vi "关键参数交互.vi"(9 "量程下拉列表":refnum<vi>, 10 "测量模式下拉列表":refnum<vi>, 11 "参数下拉列表":refnum<vi>) -> ()   [LabVIEW 2016, in "斯坦道总氮.lvlib"]
panel:
  out "总氮仪器参数":T1
  out "总磷仪器参数":T1
  out "x != y? 2":T2
  out "x != y?":T2
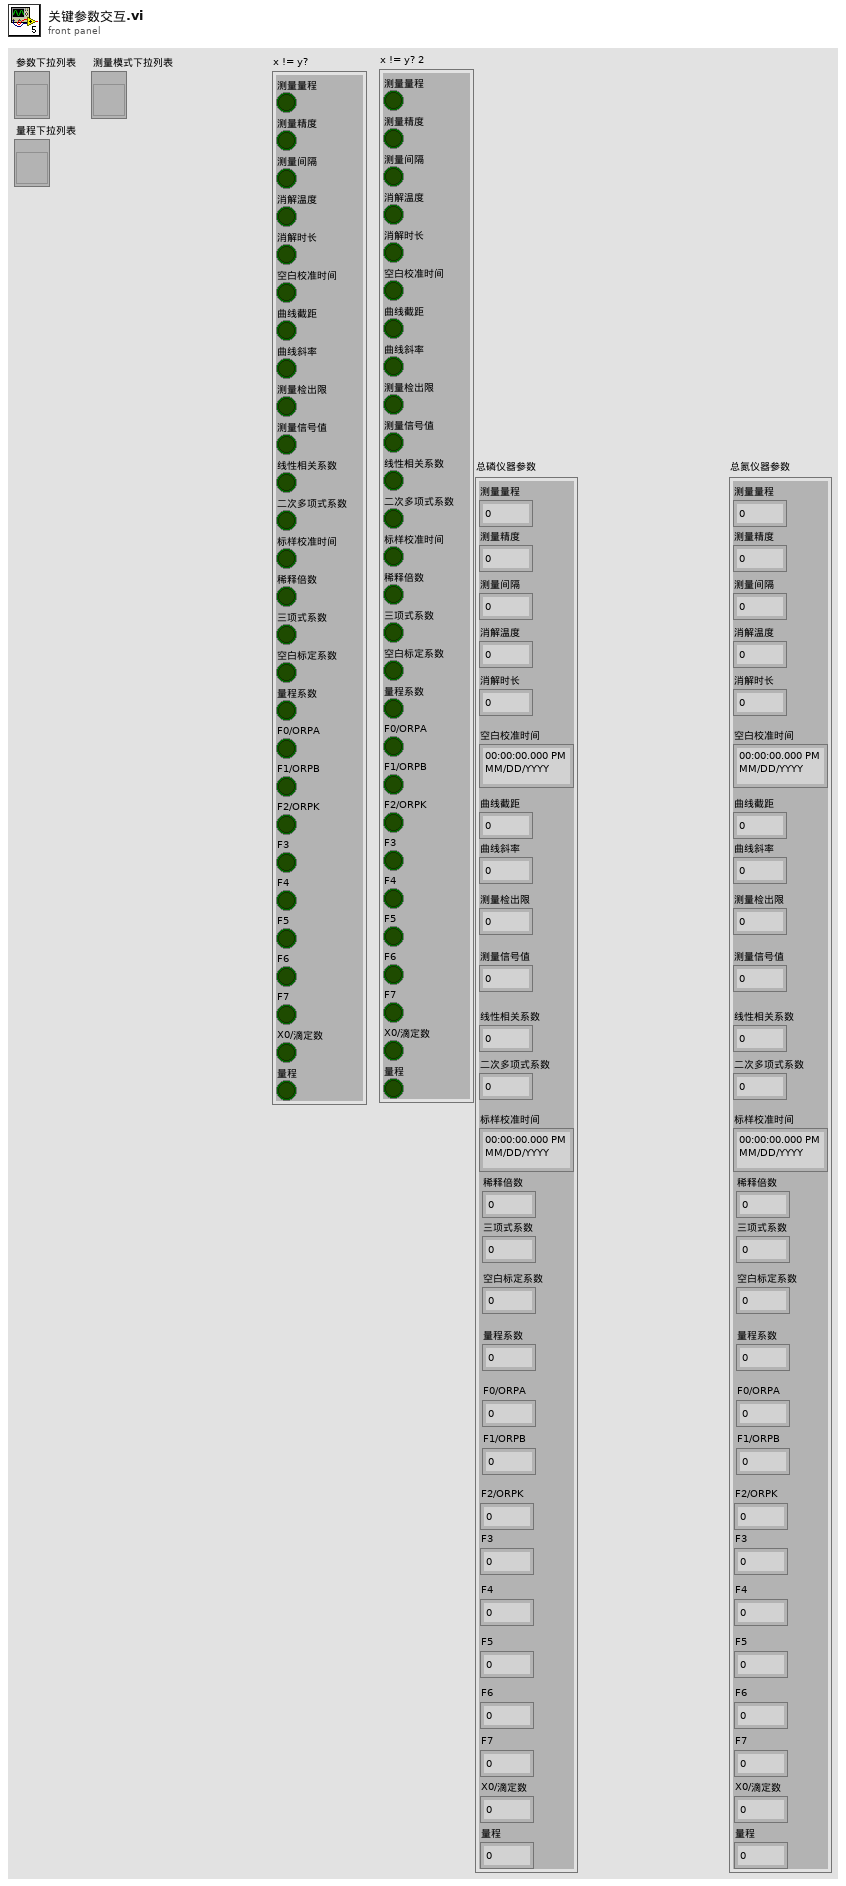
[diagram p1: front panel]
types:
  T1 = cluster{"测量量程":dbl, "测量精度":dbl, "测量间隔":dbl, "消解温度":dbl, "消解时长":dbl, "空白校准时间":timestamp, "曲线截距":dbl, "曲线斜率":dbl, "测量检出限":dbl, "测量信号值":dbl, "线性相关系数":dbl, "二次多项式系数":dbl, "标样校准时间":timestamp, "稀释倍数":dbl, "三项式系数":dbl, "空白标定系数":dbl, "量程系数":dbl, "F0/ORPA":dbl, "F1/ORPB":dbl, "F2/ORPK":dbl, "F3":dbl, "F4":dbl, "F5":dbl, "F6":dbl, "F7":dbl, "X0/滴定数":dbl, "量程":dbl}
  T2 = cluster{"测量量程":bool, "测量精度":bool, "测量间隔":bool, "消解温度":bool, "消解时长":bool, "空白校准时间":bool, "曲线截距":bool, "曲线斜率":bool, "测量检出限":bool, "测量信号值":bool, "线性相关系数":bool, "二次多项式系数":bool, "标样校准时间":bool, "稀释倍数":bool, "三项式系数":bool, "空白标定系数":bool, "量程系数":bool, "F0/ORPA":bool, "F1/ORPB":bool, "F2/ORPK":bool, "F3":bool, "F4":bool, "F5":bool, "F6":bool, "F7":bool, "X0/滴定数":bool, "量程":bool}
  T3 = cluster{"chose":string, "公式":cluster{"X^2":dbl, "X":dbl, "b":dbl}}
  T4 = cluster{"时间标识":timestamp, "设备":string, "日志信息":string, "流程参数":string}
  T5 = cluster{"[0]":bool, "[1]":bool, "[2]":bool, "[3]":bool, "[4]":bool, "[5]":bool, "[6]":bool, "[7]":bool, "[8]":bool, "[9]":bool, "[10]":bool, "[11]":bool, "[12]":bool, "[13]":bool, "[14]":bool, "[15]":bool, "[16]":bool, "[17]":bool, "[18]":bool, "[19]":bool, "[20]":bool, "[21]":bool, "[22]":bool, "[23]":bool, "[24]":bool, "[25]":bool, "[26]":bool}
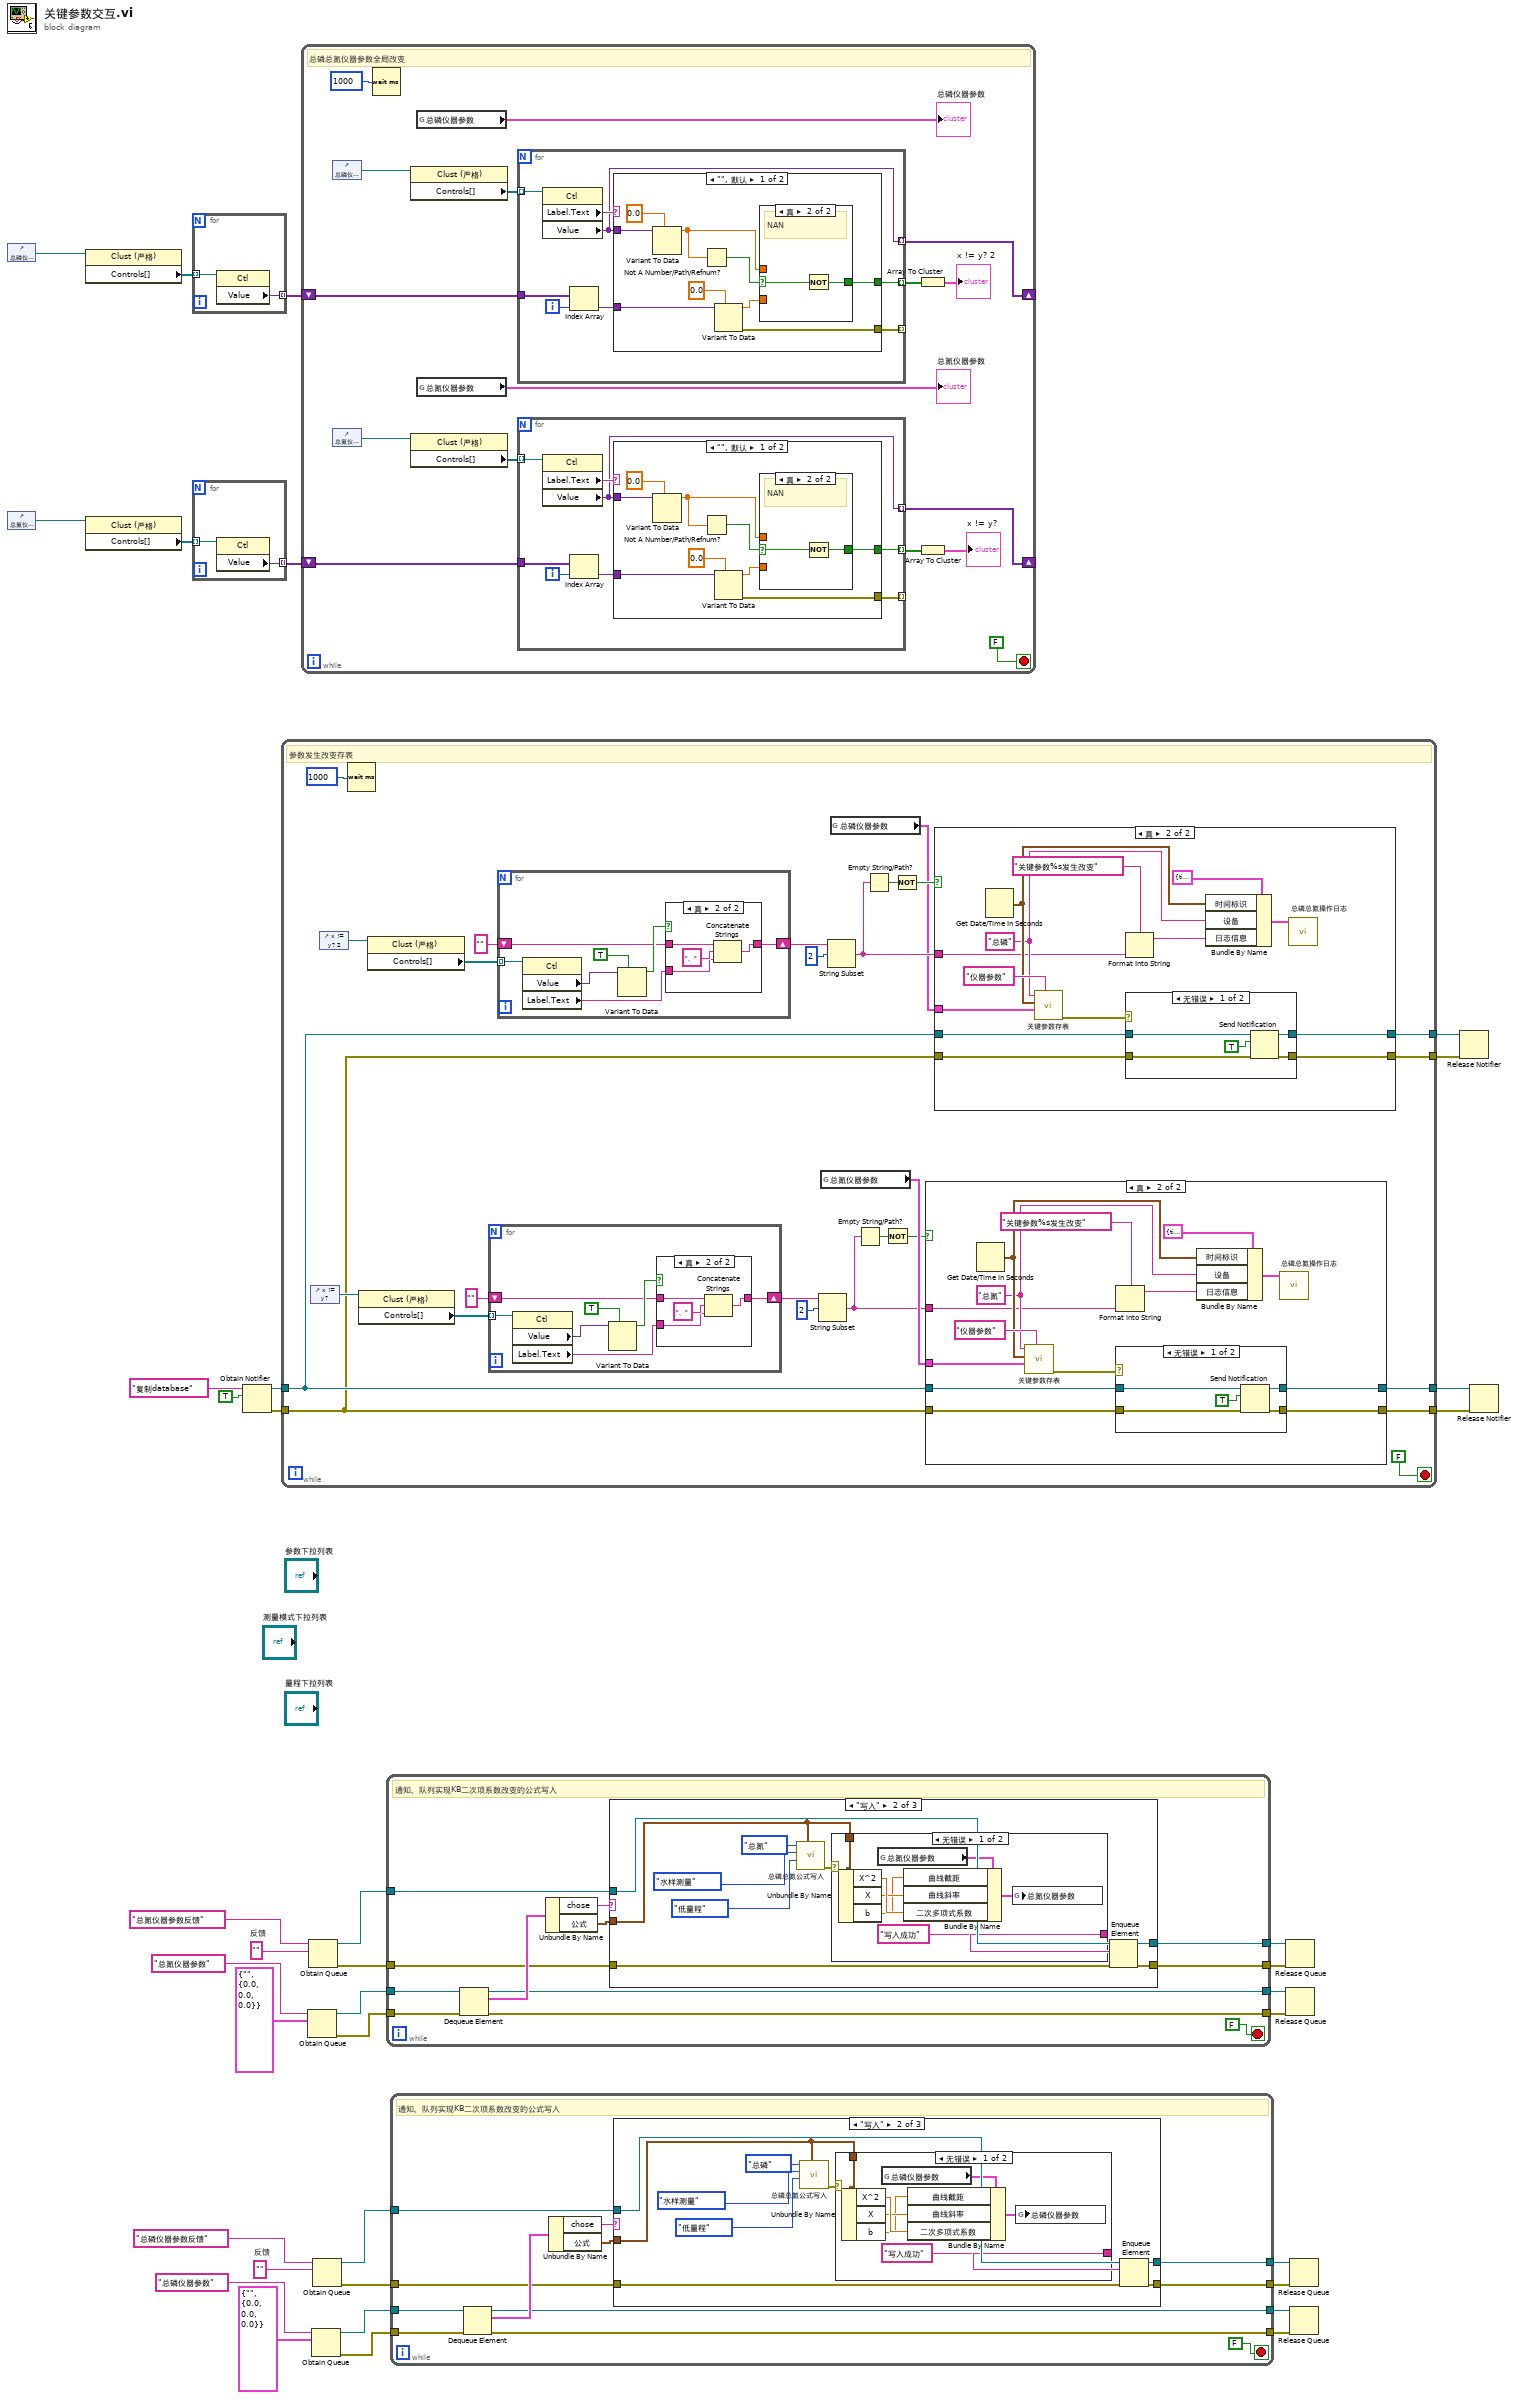
[diagram p0: block diagram]
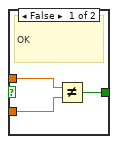
[diagram p2: hidden frame]
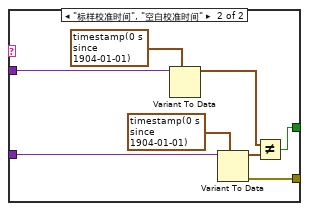
[diagram p3: hidden frame]
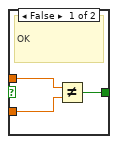
[diagram p4: hidden frame]
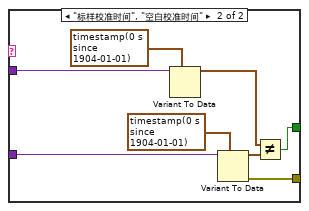
[diagram p5: hidden frame]
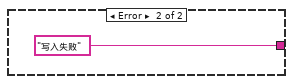
[diagram p7: hidden frame]
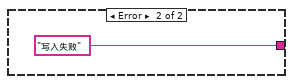
[diagram p10: hidden frame]
diagram:
  w15 = ""  # 反馈
  w32 = ""  # 反馈
  n1 = control-ref of="总磷仪器参数"() -> (w5:refnum<vi>)
  n2 = control-ref of="总氮仪器参数"() -> (w2:refnum<vi>)
  n3 = property class="Clust (严格)"(reference=w5) -> ("Controls[]"=w6:refnum<vi>[])  [unwired: 1 in, 2 out]
  n4 = property class="Clust (严格)"(reference=w2) -> ("Controls[]"=w3:refnum<vi>[])  [unwired: 1 in, 2 out]
  n5 = for {
    tunnel: w6 -> [w40] mode=indexing
    tunnel: [w39] -> w4 mode=indexing
    n6 = property class="Ctl"(reference=w40) -> ("Value"=w39:variant)  [unwired: 1 in, 2 out]
  }
  n7 = for {
    tunnel: w3 -> [w42] mode=indexing
    tunnel: [w41] -> w1 mode=indexing
    n8 = property class="Ctl"(reference=w42) -> ("Value"=w41:variant)  [unwired: 1 in, 2 out]
  }
  n9 = Obtain Notifier(name (unnamed)="复制database" ("名称（未命名）"), notification data type=TRUE) -> (notifier out=w24:refnum<notifier>, error out=w23:errorcluster)  [unwired: 2 in, 1 out]
  n10 = while {
    tunnel: w24 -> [w46]
    tunnel: w23 -> [w45]
    tunnel: [w64] -> w22
    tunnel: [w63] -> w21
    tunnel: [w44] -> w8
    tunnel: [w43] -> w7
    stop <- FALSE stop-if-true
    # "参数发生改变存表"
    n11 = control-ref of="x != y?"() -> (w66:refnum<vi>)
    n12 = control-ref of="x != y? 2"() -> (w48:refnum<vi>)
    n13 = Wait (ms)(milliseconds to wait=u32 1000 ("等待时间（毫秒）")) -> ()  [unwired: 1 out]
    n14 = property class="Clust (严格)"(reference=w66) -> ("Controls[]"=w59:refnum<vi>[])  [unwired: 1 in, 2 out]
    n15 = property class="Clust (严格)"(reference=w48) -> ("Controls[]"=w52:refnum<vi>[])  [unwired: 1 in, 2 out]
    n16 = for {
      tunnel: w59 -> [w110] mode=indexing
      shift-right: [w104] -> w61
      shift-left: "" -> [w106]
      n17 = property class="Ctl"(reference=w110) -> ("Value"=w108:variant, "Label.Text"=w105:string)  [unwired: 1 in, 2 out]
      n18 = Variant To Data(type=TRUE, Variant=w108) -> (data=w107:bool)  [unwired: 1 in, 1 out]
      n19 = case shown="真" w107 {
        tunnel: w106 -> [w111 w115]
        tunnel: w105 -> [_ w112]
        tunnel: [w111 w114] -> w104
        frame False {
        }
        frame True {
          n20 = Concatenate Strings(w115, "、", w112) -> (w114:string)
        }
      }
    }
    n21 = for {
      tunnel: w52 -> [w75] mode=indexing
      shift-right: [w69] -> w50
      shift-left: "" -> [w71]
      n22 = property class="Ctl"(reference=w75) -> ("Value"=w73:variant, "Label.Text"=w70:string)  [unwired: 1 in, 2 out]
      n23 = Variant To Data(type=TRUE, Variant=w73) -> (data=w72:bool)  [unwired: 1 in, 1 out]
      n24 = case shown="真" w72 {
        tunnel: w71 -> [w76 w80]
        tunnel: w70 -> [_ w77]
        tunnel: [w76 w79] -> w69
        frame False {
        }
        frame True {
          n25 = Concatenate Strings(w80, "、", w77) -> (w79:string)
        }
      }
    }
    n26 = String Subset(string=w61, offset (0)=2 ("偏移量(0)")) -> (substring=w56:string)  [unwired: 1 in]
    n27 = global read "总磷总氮断电保存全局变量.vi" "总氮仪器参数"() -> (w65:T1)
    n28 = String Subset(string=w50, offset (0)=2 ("偏移量(0)")) -> (substring=w55:string)  [unwired: 1 in]
    n29 = global read "总磷总氮断电保存全局变量.vi" "总磷仪器参数"() -> (w47:T1)
    n30 = Empty String/Path?(string/path=w56) -> (empty?=w58:bool)
    n31 = Empty String/Path?(string/path=w55) -> (empty?=w53:bool)
    n32 = Not(x=w58) -> (.not. x?=w57:bool)
    n33 = Not(x=w53) -> (.not. x?=w54:bool)
    n34 = case shown="真" w57 {
      tunnel: w65 -> [_ w130]
      tunnel: w56 -> [_ w124]
      tunnel: w46 -> [w117 w122]
      tunnel: w45 -> [w116 w121]
      tunnel: [w117 w119] -> w64
      tunnel: [w116 w118] -> w63
      frame False {
      }
      frame True {
        w126 = "总氮" ("仪器名称")
        n35 = Get Date/Time In Seconds() -> (seconds since 1Jan1904=w127:timestamp)
        n36 = call "关键参数存表.vi"("table"="仪器参数", "仪器参数"=w130, "datatime"=w127, "仪器名称"=w126) -> ("error out"=w120:errorcluster)  [unwired: 7 in]
        n37 = Format Into String(format string="关键参数%s发生改变" ("格式字符串"), w124) -> (resulting string=w123:string)  [unwired: 2 in, 1 out]
        n38 = case shown="无错误" w120 {
          tunnel: w122 -> [w136 w138]
          tunnel: w121 -> [w135 w137]
          tunnel: [w133 w138] -> w119
          tunnel: [w132 w137] -> w118
          frame No Error {
            n39 = Send Notification(notification=TRUE ("通知"), notifier=w136, error in (no error)=w135) -> (notifier out=w133:refnum<notifier>, error out=w132:errorcluster)
          }
          frame Error {
          }
        }
        n40 = Bundle By Name(cluster=T4 {"时间标识"=timestamp(0 s since 1904-01-01), "设备"="", "日志信息"="", "流程参数"=""} ("data in"), "时间标识"=w127, "设备"=w126, "日志信息"=w123) -> (w128:T4)
        n41 = call "总磷总氮操作日志.vi"("data in"=w128) -> ()  [unwired: 11 in]
      }
    }
    n42 = case shown="真" w54 {
      tunnel: w47 -> [_ w95]
      tunnel: w55 -> [_ w89]
      tunnel: w46 -> [w82 w87]
      tunnel: w45 -> [w81 w86]
      tunnel: [w82 w84] -> w44
      tunnel: [w81 w83] -> w43
      frame False {
      }
      frame True {
        w91 = "总磷" ("仪器名称")
        n43 = Get Date/Time In Seconds() -> (seconds since 1Jan1904=w92:timestamp)
        n44 = call "关键参数存表.vi"("table"="仪器参数", "仪器参数"=w95, "datatime"=w92, "仪器名称"=w91) -> ("error out"=w85:errorcluster)  [unwired: 7 in]
        n45 = Format Into String(format string="关键参数%s发生改变" ("格式字符串"), w89) -> (resulting string=w88:string)  [unwired: 2 in, 1 out]
        n46 = case shown="无错误" w85 {
          tunnel: w87 -> [w101 w103]
          tunnel: w86 -> [w100 w102]
          tunnel: [w98 w103] -> w84
          tunnel: [w97 w102] -> w83
          frame No Error {
            n47 = Send Notification(notification=TRUE ("通知"), notifier=w101, error in (no error)=w100) -> (notifier out=w98:refnum<notifier>, error out=w97:errorcluster)
          }
          frame Error {
          }
        }
        n48 = Bundle By Name(cluster=T4 {"时间标识"=timestamp(0 s since 1904-01-01), "设备"="", "日志信息"="", "流程参数"=""} ("data in"), "时间标识"=w92, "设备"=w91, "日志信息"=w88) -> (w93:T4)
        n49 = call "总磷总氮操作日志.vi"("data in"=w93) -> ()  [unwired: 11 in]
      }
    }
  }
  n50 = while {
    shift-right: [w148] -> _
    shift-left: w4 -> [w149]
    shift-right: [w139] -> _
    shift-left: w1 -> [w140]
    stop <- FALSE stop-if-true
    # "总磷总氮仪器参数全局改变"
    n51 = control-ref of="总磷仪器参数"() -> (w154:refnum<vi>)
    n52 = control-ref of="总氮仪器参数"() -> (w141:refnum<vi>)
    n53 = Wait (ms)(milliseconds to wait=u32 1000 ("等待时间（毫秒）")) -> ()  [unwired: 1 out]
    n54 = property class="Clust (严格)"(reference=w154) -> ("Controls[]"=w151:refnum<vi>[])  [unwired: 1 in, 2 out]
    n55 = property class="Clust (严格)"(reference=w141) -> ("Controls[]"=w143:refnum<vi>[])  [unwired: 1 in, 2 out]
    n56 = global read "总磷总氮断电保存全局变量.vi" "总磷仪器参数"() -> (→"总磷仪器参数":T1)
    n57 = global read "总磷总氮断电保存全局变量.vi" "总氮仪器参数"() -> (→"总氮仪器参数":T1)
    n58 = for {
      tunnel: w151 -> [w192] mode=indexing
      tunnel: [w190] -> w150 mode=indexing
      tunnel: [w188] -> _ mode=indexing
      tunnel: w149 -> [w187]
      tunnel: [w189] -> w148 mode=indexing
      i -> [w186]
      n59 = property class="Ctl"(reference=w192) -> ("Label.Text"=w191:string, "Value"=w189:variant)  [unwired: 1 in, 2 out]
      n60 = Index Array(array=w187, index=w186) -> (element=w185:variant)
      n61 = case shown="\"\", 默认" w191 {
        tunnel: w189 -> [w201 w214]
        tunnel: [w195 w208] -> w190
        tunnel: w185 -> [w198 w211]
        tunnel: [w197 w207] -> w188
        frame "", Default {
          n62 = Variant To Data(type=0.0 ("测量检出限"), Variant=w201) -> (data=w194:dbl)  [unwired: 1 in, 1 out]
          n63 = Not A Number/Path/Refnum?(number/path/refnum=w194) -> (NaN/Path/Refnum?=w196:bool)
          n64 = Variant To Data(type=0.0 ("测量检出限"), Variant=w198) -> (data=w193:dbl, error out=w197:errorcluster)  [unwired: 1 in]
          n65 = case shown="真" w196 {
            selector: w196 -> [_ w206]
            tunnel: [w202 w205] -> w195
            tunnel: w194 -> [w204 _]
            tunnel: w193 -> [w203 _]
            frame False {
              # "OK"
              n66 = Not Equal?(x=w204, y=w203) -> (x != y?=w202:bool)
            }
            frame True {
              # "NAN"
              n67 = Not(x=w206) -> (.not. x?=w205:bool)
            }
          }
        }
        frame "标样校准时间", "空白校准时间" {
          n68 = Variant To Data(type=timestamp(0 s since 1904-01-01), Variant=w214) -> (data=w210:timestamp)  [unwired: 1 in, 1 out]
          n69 = Variant To Data(type=timestamp(0 s since 1904-01-01), Variant=w211) -> (data=w209:timestamp, error out=w207:errorcluster)  [unwired: 1 in]
          n70 = Not Equal?(x=w210, y=w209) -> (x != y?=w208:bool)
        }
      }
    }
    n71 = for {
      tunnel: w143 -> [w162] mode=indexing
      tunnel: [w160] -> w144 mode=indexing
      tunnel: [w158] -> _ mode=indexing
      tunnel: w140 -> [w157]
      tunnel: [w159] -> w139 mode=indexing
      i -> [w156]
      n72 = property class="Ctl"(reference=w162) -> ("Label.Text"=w161:string, "Value"=w159:variant)  [unwired: 1 in, 2 out]
      n73 = Index Array(array=w157, index=w156) -> (element=w155:variant)
      n74 = case shown="\"\", 默认" w161 {
        tunnel: w159 -> [w171 w184]
        tunnel: [w165 w178] -> w160
        tunnel: w155 -> [w168 w181]
        tunnel: [w167 w177] -> w158
        frame "", Default {
          n75 = Variant To Data(type=0.0 ("测量检出限"), Variant=w171) -> (data=w164:dbl)  [unwired: 1 in, 1 out]
          n76 = Not A Number/Path/Refnum?(number/path/refnum=w164) -> (NaN/Path/Refnum?=w166:bool)
          n77 = Variant To Data(type=0.0 ("测量检出限"), Variant=w168) -> (data=w163:dbl, error out=w167:errorcluster)  [unwired: 1 in]
          n78 = case shown="真" w166 {
            selector: w166 -> [_ w176]
            tunnel: [w172 w175] -> w165
            tunnel: w164 -> [w174 _]
            tunnel: w163 -> [w173 _]
            frame False {
              # "OK"
              n79 = Not Equal?(x=w174, y=w173) -> (x != y?=w172:bool)
            }
            frame True {
              # "NAN"
              n80 = Not(x=w176) -> (.not. x?=w175:bool)
            }
          }
        }
        frame "标样校准时间", "空白校准时间" {
          n81 = Variant To Data(type=timestamp(0 s since 1904-01-01), Variant=w184) -> (data=w180:timestamp)  [unwired: 1 in, 1 out]
          n82 = Variant To Data(type=timestamp(0 s since 1904-01-01), Variant=w181) -> (data=w179:timestamp, error out=w177:errorcluster)  [unwired: 1 in]
          n83 = Not Equal?(x=w180, y=w179) -> (x != y?=w178:bool)
        }
      }
    }
    n84 = Array To Cluster(array=w150) -> (cluster=→"x != y? 2":T5)
    n85 = Array To Cluster(array=w144) -> (cluster=→"x != y?":T5)
  }
  n86 = Obtain Queue(name (unnamed)="总氮仪器参数" ("名称（未命名）"), element data type=T3 {"chose"="", "公式"={"X^2"=0.0, "X"=0.0, "b"=0.0}}) -> (queue out=w28:refnum<queue>, error out=w27:errorcluster)  [unwired: 3 in, 1 out]
  n87 = Obtain Queue(name (unnamed)="总氮仪器参数反馈" ("名称（未命名）"), element data type=w32) -> (queue out=w33:refnum<queue>, error out=w31:errorcluster)  [unwired: 3 in, 1 out]
  n88 = Obtain Queue(name (unnamed)="总磷仪器参数" ("名称（未命名）"), element data type=T3 {"chose"="", "公式"={"X^2"=0.0, "X"=0.0, "b"=0.0}}) -> (queue out=w19:refnum<queue>, error out=w20:errorcluster)  [unwired: 3 in, 1 out]
  n89 = Obtain Queue(name (unnamed)="总磷仪器参数反馈" ("名称（未命名）"), element data type=w15) -> (queue out=w14:refnum<queue>, error out=w16:errorcluster)  [unwired: 3 in, 1 out]
  n90 = while {
    tunnel: w28 -> [w225]
    tunnel: w27 -> [w224]
    tunnel: [w216] -> w36
    tunnel: [w215] -> w35
    tunnel: w33 -> [w220]
    tunnel: w31 -> [w219]
    tunnel: [w218] -> w30
    tunnel: [w217] -> w29
    stop <- FALSE stop-if-true
    # "通知、队列实现KB二次项系数改变的公式写入"
    n91 = Dequeue Element(queue=w225, error in (no error)=w224) -> (queue out=w216:refnum<queue>, element=w223:T3, error out=w215:errorcluster)  [unwired: 1 in, 1 out]
    n92 = Unbundle By Name(w223) -> ("chose"=w222:string, "公式"=w221:cluster{"X^2":dbl, "X":dbl, "b":dbl})
    n93 = case shown="\"写入\"" w222 {
      tunnel: w221 -> [_ w232 _]
      tunnel: w220 -> [w228 w237 w248]
      tunnel: w219 -> [w227 w235 w247]
      tunnel: [w228 w234 w248] -> w218
      tunnel: [w227 w233 w247] -> w217
      frame "假", Default {
      }
      frame "写入" {
        n94 = call "总磷总氮公式写入.vi"("公式"=w232, "量程"=enum16{"低量程", "高量程"}."低量程", "测量模式"=enum16{"水样测量", "零点核查", "跨度核查", "标样核查", "加标回收"}."水样测量", "测量参数"=enum16{"COD", "氨氮", "总氮", "总磷"}."总氮") -> ("error out"=w238:errorcluster)  [unwired: 7 in]
        n95 = case shown="无错误" w238 {
          tunnel: ["写入成功" ("消息") "写入失败" ("消息")] -> w236
          tunnel: w232 -> [w242 _]
          frame No Error {
            n96 = Unbundle By Name(w242) -> ("X^2"=w241:dbl, "X"=w240:dbl, "b"=w239:dbl)
            n97 = global read "总磷总氮断电保存全局变量.vi" "总氮仪器参数"() -> (w243:T1)
            n98 = Bundle By Name(cluster=w243, "曲线截距"=w239, "曲线斜率"=w240, "二次多项式系数"=w241) -> (w244:T1)
            n99 = global write "总磷总氮断电保存全局变量.vi" "总氮仪器参数"(w244) -> ()
          }
          frame Error {
          }
        }
        n100 = Enqueue Element(queue=w237, element=w236, error in (no error)=w235) -> (queue out=w234:refnum<queue>, error out=w233:errorcluster)  [unwired: 1 in, 1 out]
      }
      frame "读取" {
      }
    }
  }
  n101 = while {
    tunnel: w19 -> [w259]
    tunnel: w20 -> [w258]
    tunnel: [w250] -> w11
    tunnel: [w249] -> w12
    tunnel: w14 -> [w254]
    tunnel: w16 -> [w253]
    tunnel: [w252] -> w17
    tunnel: [w251] -> w18
    stop <- FALSE stop-if-true
    # "通知、队列实现KB二次项系数改变的公式写入"
    n102 = Dequeue Element(queue=w259, error in (no error)=w258) -> (queue out=w250:refnum<queue>, element=w257:T3, error out=w249:errorcluster)  [unwired: 1 in, 1 out]
    n103 = Unbundle By Name(w257) -> ("chose"=w256:string, "公式"=w255:cluster{"X^2":dbl, "X":dbl, "b":dbl})
    n104 = case shown="\"写入\"" w256 {
      tunnel: w255 -> [_ w266 _]
      tunnel: w254 -> [w262 w271 w282]
      tunnel: w253 -> [w261 w269 w281]
      tunnel: [w262 w268 w282] -> w252
      tunnel: [w261 w267 w281] -> w251
      frame "假", Default {
      }
      frame "写入" {
        n105 = call "总磷总氮公式写入.vi"("公式"=w266, "量程"=enum16{"低量程", "高量程"}."低量程", "测量模式"=enum16{"水样测量", "零点核查", "跨度核查", "标样核查", "加标回收"}."水样测量", "测量参数"=enum16{"COD", "氨氮", "总氮", "总磷"}."总磷") -> ("error out"=w272:errorcluster)  [unwired: 7 in]
        n106 = case shown="无错误" w272 {
          tunnel: ["写入成功" ("消息") "写入失败" ("消息")] -> w270
          tunnel: w266 -> [w276 _]
          frame No Error {
            n107 = Unbundle By Name(w276) -> ("X^2"=w275:dbl, "X"=w274:dbl, "b"=w273:dbl)
            n108 = global read "总磷总氮断电保存全局变量.vi" "总磷仪器参数"() -> (w277:T1)
            n109 = Bundle By Name(cluster=w277, "曲线截距"=w273, "曲线斜率"=w274, "二次多项式系数"=w275) -> (w278:T1)
            n110 = global write "总磷总氮断电保存全局变量.vi" "总磷仪器参数"(w278) -> ()
          }
          frame Error {
          }
        }
        n111 = Enqueue Element(queue=w271, element=w270, error in (no error)=w269) -> (queue out=w268:refnum<queue>, error out=w267:errorcluster)  [unwired: 1 in, 1 out]
      }
      frame "读取" {
      }
    }
  }
  n112 = Release Queue(queue=w30, error in (no error)=w29) -> ()  [unwired: 1 in, 3 out]
  n113 = Release Queue(queue=w36, error in (no error)=w35) -> ()  [unwired: 1 in, 3 out]
  n114 = Release Queue(queue=w17, error in (no error)=w18) -> ()  [unwired: 1 in, 3 out]
  n115 = Release Queue(queue=w11, error in (no error)=w12) -> ()  [unwired: 1 in, 3 out]
  n116 = Release Notifier(notifier=w8, error in (no error)=w7) -> ()  [unwired: 1 in, 3 out]
  n117 = Release Notifier(notifier=w22, error in (no error)=w21) -> ()  [unwired: 1 in, 3 out]
